vi "AES APU Acceleration To Increment Rate.vi"(7 "FPGA clock (40M)":dbl=40000000.0, 10 "acceleration (RPM/sec)":dbl) -> (3 "increment rate":fxp<+/-,47,-4> format="%.50g")   [LabVIEW 2010, in "AES.lvlib" / "AES RT.lvlib"]
uses:
  AES RT.lvlib
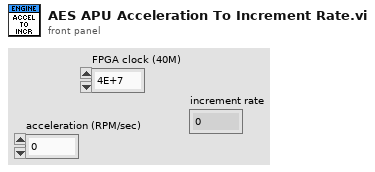
[diagram p1: front panel]
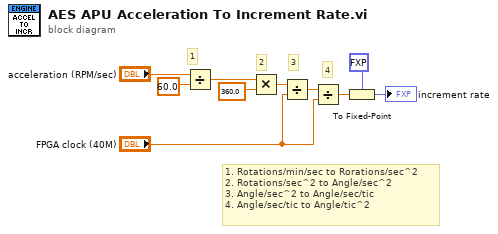
[diagram p0: block diagram]
diagram:
  # "1. Rotations/min/sec to Rorations/sec^2\n2. Rotations/sec^2 to Angle/sec^2\n3. Angle/sec^2 to Angle/sec/tic\n4. Angle/sec/tic to Angle/tic^2"
  # "4"
  # "3"
  # "2"
  # "1"
  n1 = Divide(x="acceleration (RPM/sec)", y=60.0) -> (x/y=w6:dbl)
  n2 = Multiply(x=w6, y=360.0) -> (x*y=w4:dbl)
  n3 = Divide(x=w4, y="FPGA clock (40M)") -> (x/y=w3:dbl)
  n4 = Divide(x=w3, y="FPGA clock (40M)") -> (x/y=w1:dbl)
  n5 = To Fixed-Point(fixed-point type=fxp<+/-,47,-4> 0.0, number=w1) -> (fixed-point=→"increment rate":fxp<+/-,47,-4>)
